vi "PKG_IMC_SetEncpMode.vi"(7 "axis":i32, 9 "dir":i32, 10 "mode":i32, 11 "handle":u32) -> (2 "function return":i32, 3 "handle out":u32)   [LabVIEW 2018, in "IMC_Pkg4xxx.lvlib"]
doc: "PKG_IMC_SetEncpMode(IMC_HANDLE handle, int mode, int dir, int axis);"
uses:
  IMC_Pkg4xxx.lvlib
  IMC_Pkg4xxx.dll
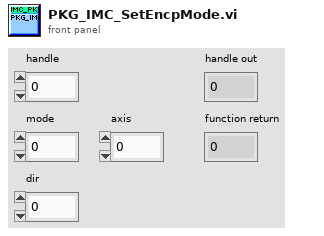
[diagram p1: front panel]
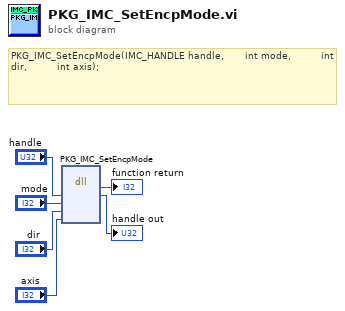
[diagram p0: block diagram]
diagram:
  # "PKG_IMC_SetEncpMode(IMC_HANDLE handle, \t\t\t\t\t\tint mode, \t\t\t\t\t\t\t\t\tint dir, \t\t\t\t\t\t\t\t\tint axis);"
  n1 = dll-call lib="PTH2\\abs D做的项目航天测量驱动电机IMCAppincLabview32\nIMC_Pkg4xxx.*" fn="PKG_IMC_SetEncpMode"("handle"="handle", "mode"="mode", "dir"="dir", "axis"="axis") -> (→"function return":i32, "handle"=→"handle out":u32)  [unwired: 6 in, 2 out]
